vi "Facade.vi"(0 "Data In":T4 caption="数据输入", 2 "Display State In":T2 caption="显示状态输入", 3 "Container State":T3 caption="容器状态") -> (6 "Data Out":T4 caption="数据输出", 7 "Display State Out":T2 caption="显示状态输出", 8 "Action":T1 caption="动作")   [LabVIEW 2016, in "GradChangeColorBar.xctl"]
uses:
  GradChangeColorBar.xctl
  Data.ctl
  <vilib>/_xctls/Container State.ctl
  State.ctl
  <vilib>/_xctls/Action.ctl
  <vilib>/picture/picture.llb/Draw True-Color Pixmap.vi
  <vilib>/_xctls/XControlSupport.lvlib
panel:
  out "GradChangeColorBar":picture
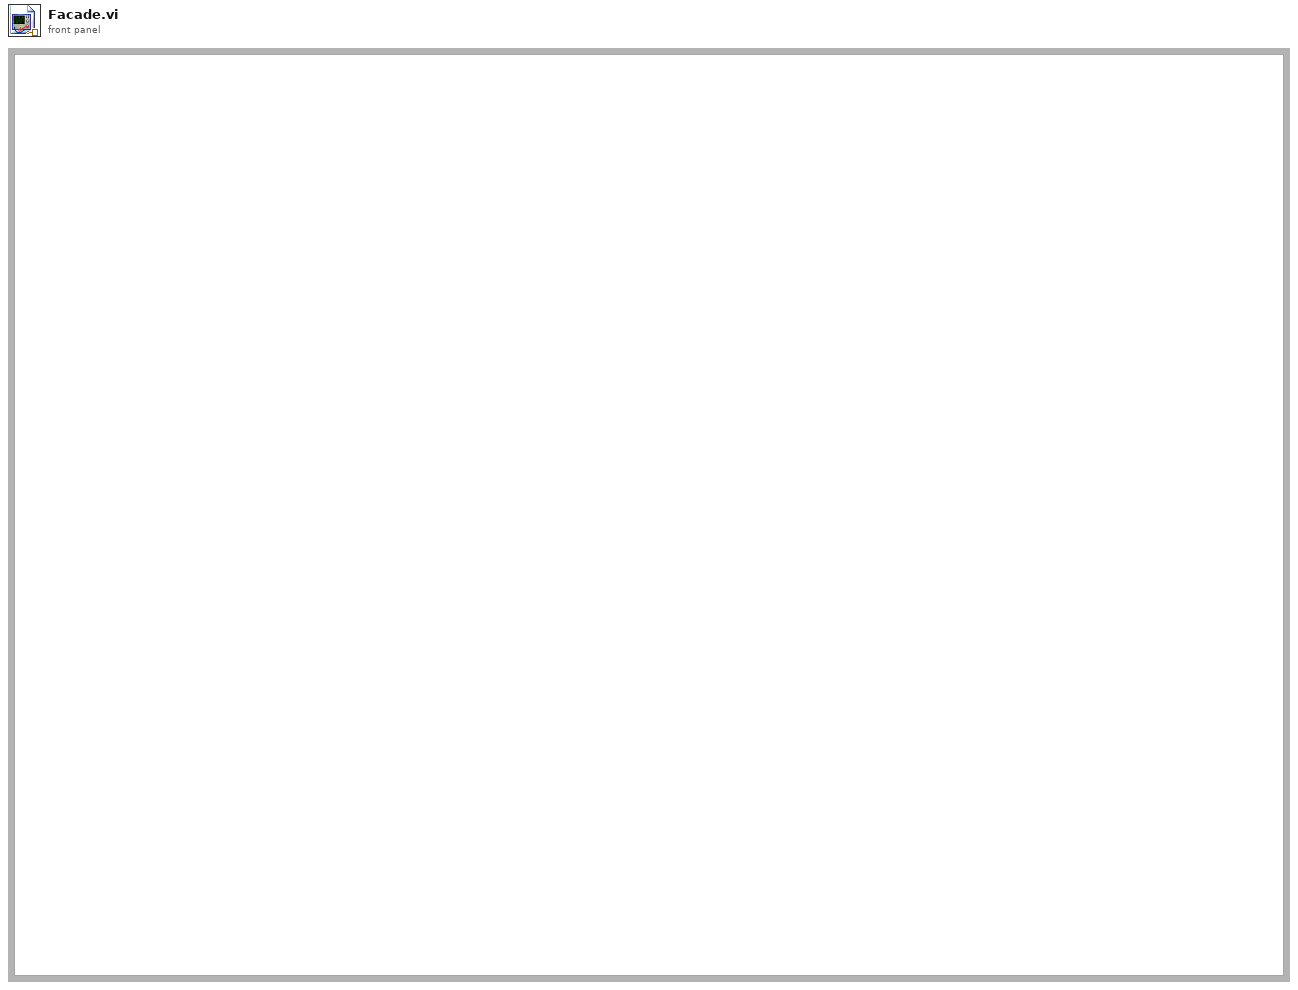
[diagram p1: front panel]
types:
  T1 = typedef "XControlSupport.lvlib/Action.ctl" = cluster{"Data Changed?":bool, "State Changed?":bool, "Action Name":string}
  T2 = typedef "GradChangeColorBar.xctl/State.ctl" = cluster{"Numeric":dbl}
  T3 = typedef "XControlSupport.lvlib/Container State.ctl" = cluster{"Indicator?":bool, "Run Mode?":bool, " Refnum":refnum<vi>}
  T4 = typedef "GradChangeColorBar.xctl/Data.ctl" = cluster{cluster{dbl, "R":dbl}[], cluster{dbl, "G":dbl}[], cluster{dbl, "B":dbl}[]}
  T5 = typedef "LVBoundsTypeDef.ctl" = cluster{"Width":u32, "Height":u32}
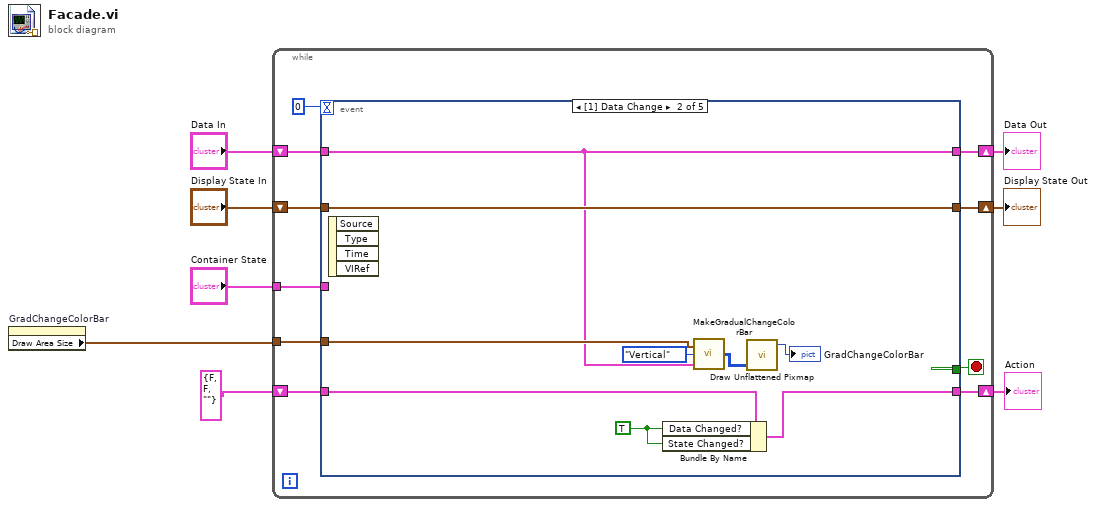
[diagram p0: block diagram]
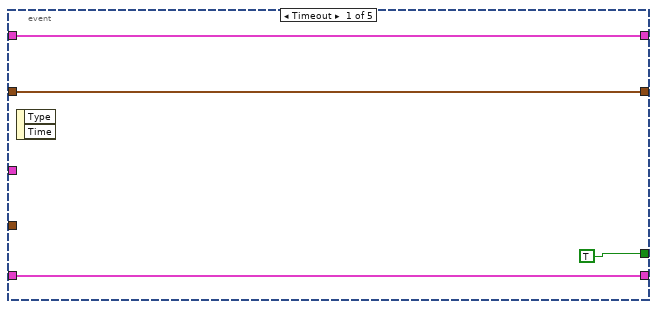
[diagram p2: hidden frame]
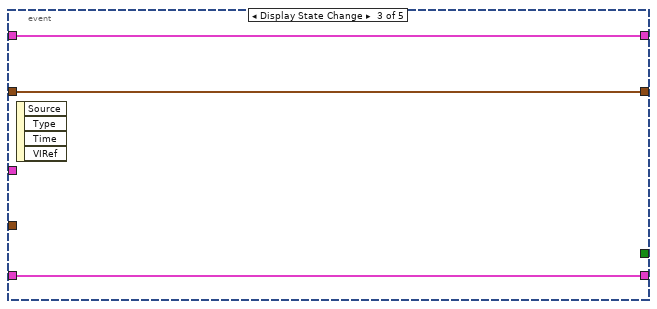
[diagram p3: hidden frame]
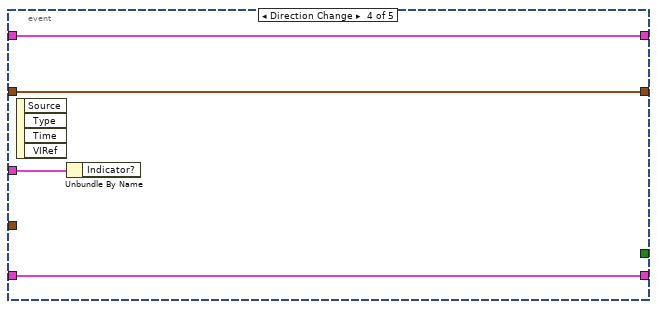
[diagram p4: hidden frame]
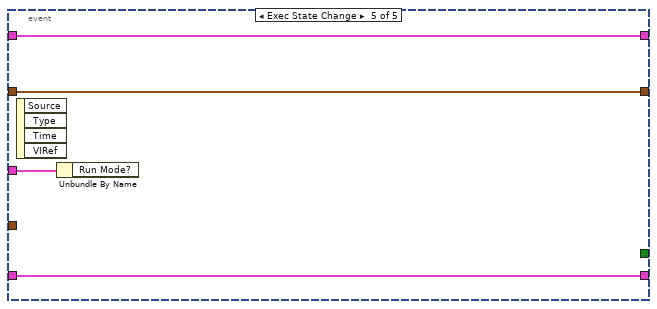
[diagram p5: hidden frame]
diagram:
  n1 = property on="GradChangeColorBar" class="Pict"() -> ("Draw Area Size"=w1:T5)  [unwired: 2 in, 2 out]
  n2 = while {
    shift-right: [w17] -> w5
    shift-left: "Display State In" -> [w18]
    tunnel: "Container State" -> [w14]
    shift-right: [w12] -> w8
    shift-left: "Data In" -> [w13]
    shift-right: [w10] -> w3
    shift-left: T1 {"Data Changed?"=FALSE, "State Changed?"=FALSE, "Action Name"=""} ("Action") -> [w11]
    tunnel: w1 -> [w9]
    stop <- w16 stop-if-true
    n3 = event shown="[1] Data Change" {
      selector: _ -> [_ _ _ _ _]
      dyn-events: _ -> [_ _ _ _ _]
      timeout: 0 -> [_ _ _ _ _]
      tunnel: w18 -> [w20 w31 w34 w37 w41]
      tunnel: [w20 w31 w34 w37 w41] -> w17
      tunnel: [TRUE _ _ _ _] -> w16
      tunnel: w14 -> [_ _ _ w38 w42]
      tunnel: w13 -> [w19 w26 w33 w36 w40]
      tunnel: [w19 w26 w33 w36 w40] -> w12
      tunnel: [w21 w29 w32 w35 w39] -> w10
      tunnel: w11 -> [w21 w30 w32 w35 w39]
      tunnel: w9 -> [_ w27 _ _ _]
      event Timeout {
        n4 = event-data() -> ()  [unwired: 3 out]
      }
      event Data Change {
        w28 = TRUE ("Data Changed?")
        n5 = event-data() -> ()  [unwired: 5 out]
        n6 = Bundle By Name(cluster=w30, "Data Changed?"=w28, "State Changed?"=w28) -> (w29:T1)
        n7 = call "MakeGradualChangeColorBar.vi"("FalseColorData"=w26, "Direction"=enum16{"Horizontal", "Vertical"}."Vertical", "GradualChangeColorBar Size"=w27) -> ("GradualChangeColorBarPicDat"=w24:u32[][])
        n8 = call-poly <vilib>:"Draw Unflattened Pixmap.vi"("data (RGB format)"=w24) -> ("new picture"=→"GradChangeColorBar":picture)  [unwired: 3 in, 5 out]
      }
      event Display State Change {
        n9 = event-data() -> ()  [unwired: 5 out]
      }
      event Direction Change {
        n10 = event-data() -> ()  [unwired: 5 out]
        n11 = Unbundle By Name(w38) -> ()  [unwired: 1 out]
      }
      event Exec State Change {
        n12 = event-data() -> ()  [unwired: 5 out]
        n13 = Unbundle By Name(w42) -> ()  [unwired: 1 out]
      }
    }
  }
  "Display State Out" <- w5
  "Data Out" <- w8
  "Action" <- w3
